vi "Program02.vi"() -> ()   [LabVIEW 2020]
panel:
  out "zewnetrzny":i32
  out "wewnetrzny":i32
  out "Array":i32[](array[numeric])
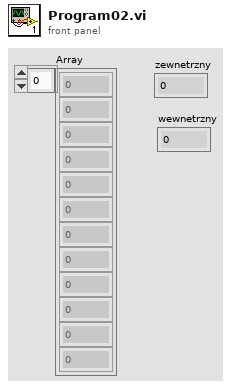
[diagram p1: front panel]
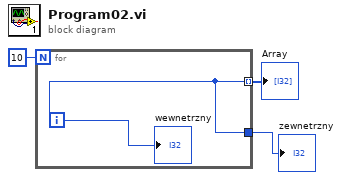
[diagram p0: block diagram]
diagram:
  n1 = for {
    N: 10 -> [_]
    tunnel: [w4] -> w2 mode=indexing
    tunnel: [w4] -> w1
    i -> [w4]
    "wewnetrzny" <- w4
  }
  "Array" <- w2
  "zewnetrzny" <- w1
